vi "KE6221 -- Set Output Response.vi"(0 "Resource In":refnum<visa-resource-name>, 1 "Check For SCPI Errors? (T)":bool=TRUE, 7 "KE6221 Output Response":T1=enum."Slow", 11 "error in (no error)":errorcluster) -> (4 "Resource Out (dupl)":refnum<visa-resource-name>, 15 "error out":errorcluster)   [LabVIEW 2013, in "Keithly user program.lvlib"]
doc: "Sets the output response speed for the 6221. For the 'Fast' selection, the output bandwidth increases to 1MHz. For the 'Slow' selection, the 6221 behaves the same as the 6220."
uses:
  Keithly user program.lvlib
  Typedefs/KE6221 -- Output Response.ctl
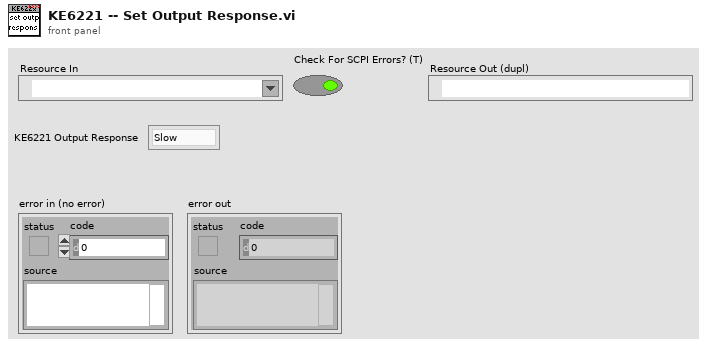
[diagram p1: front panel]
types:
  T1 = typedef "Keithly user program.lvlib/KE6221 -- Output Response.ctl" = enum16{"Fast", "Slow"}
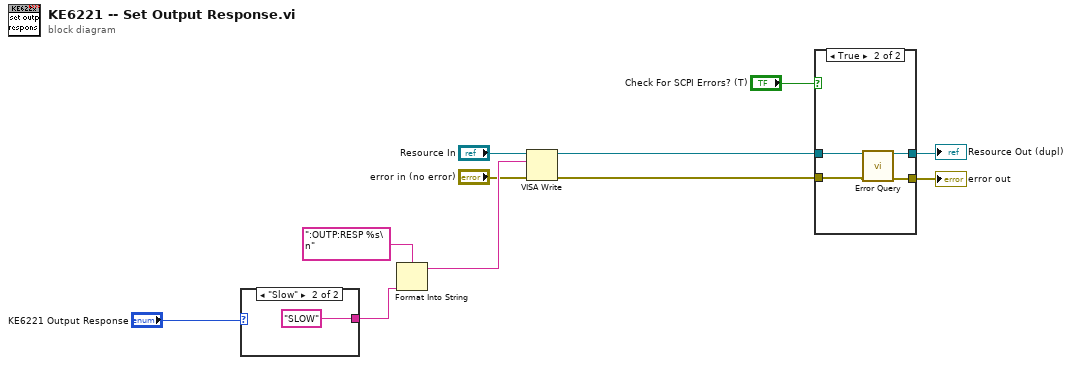
[diagram p0: block diagram]
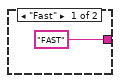
[diagram p2: hidden frame]
diagram:
  n1 = case shown="\"Slow\"" "KE6221 Output Response" {
    tunnel: ["FAST" "SLOW"] -> w2
    frame "Fast" {
    }
    frame "Slow" {
    }
  }
  n2 = Format Into String(format string=":OUTP:RESP %s\n", w2) -> (resulting string=w9:string)  [unwired: 2 in, 1 out]
  n3 = VISA Write(VISA resource name="Resource In", write buffer=w9, error in (no error)="error in (no error)") -> (VISA resource name out=w6:refnum<visa-resource-name>, error out=w5:errorcluster)  [unwired: 1 out]
  n4 = case shown="True" "Check For SCPI Errors? (T)" {
    tunnel: w6 -> [w15 w18]
    tunnel: w5 -> [w14 w17]
    tunnel: [w14 w16] -> w3
    tunnel: [w15 w19] -> w4
    frame False {
    }
    frame True {
      n5 = call "Error Query.vi"("VISA Resource In"=w18, "error in (no error)"=w17) -> ("VISA Resource Out (dupl)"=w19:refnum<visa-resource-name>, "error out"=w16:errorcluster)  [unwired: 10 in, 2 out]
    }
  }
  "Resource Out (dupl)" <- w4
  "error out" <- w3
